vi "gu_list_folder.vi"(8 "error in":errorcluster, 10 "Encoded Match":T1, 11 "Encoded String":T1) -> (0 "error out":errorcluster, 2 "Encoded Folders":T1[](array[typedef]), 3 "Encoded Files":T1[](array[typedef]))   [LabVIEW 2020, in "G-Unicode.lvlib"]
uses:
  G-Unicode.lvlib
  Types/Encoded UTF-8 String.ctl
  lib/g_unicode_32.dll
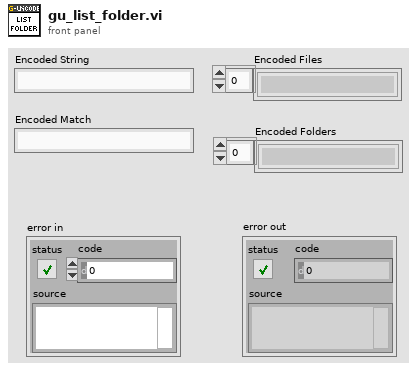
[diagram p1: front panel]
types:
  T1 = typedef "G-Unicode.lvlib/Encoded UTF-8 String.ctl" = string
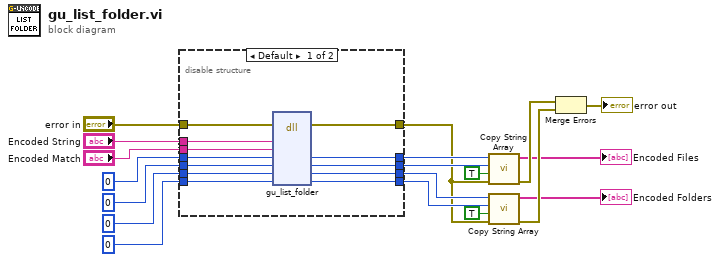
[diagram p0: block diagram]
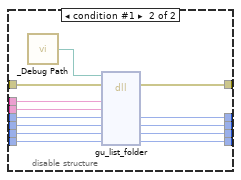
[diagram p2: hidden frame]
diagram:
  n1 = disable-structure shown="Default" {
    disable-tunnel: "Encoded String" -> [w31 w44]
    disable-tunnel: "error in" -> [w30 w43]
    disable-tunnel: [w29 w42] -> w9
    disable-tunnel: i64 0 ("files") -> [w28 w41]
    disable-tunnel: 0 ("num_files") -> [w27 w40]
    disable-tunnel: i64 0 ("folders") -> [w26 w39]
    disable-tunnel: 0 ("num_folders") -> [w25 w38]
    disable-tunnel: [w24 w37] -> w15
    disable-tunnel: [w23 w36] -> w14
    disable-tunnel: [w22 w35] -> w13
    disable-tunnel: [w21 w34] -> w12
    disable-tunnel: "Encoded Match" -> [w20 w32]
    frame condition #0 (active) {
      n2 = dll-call lib="C:/github/dataflowg/g-unicode/src/LabVIEW/G-Unicode/lib/g_unicode_*.*" fn="gu_list_folder"(error in=w30, "path"=w31, "match"=w20, "files"=w28, "num_files"=w27, "folders"=w26, "num_folders"=w25) -> (error out=w29:errorcluster, "files"=w24:i64, "num_files"=w23:i32, "folders"=w22:i64, "num_folders"=w21:i32)  [unwired: 5 in, 1 out]
    }
    frame condition #1 {
      n3 = call "_Debug Path.vi"() -> ("Debug Path"=w33:path)
      n4 = dll-call lib="?" fn="gu_list_folder"(path in=w33, error in=w43, "path"=w44, "match"=w32, "files"=w41, "num_files"=w40, "folders"=w39, "num_folders"=w38) -> (error out=w42:errorcluster, "files"=w37:i64, "num_files"=w36:i32, "folders"=w35:i64, "num_folders"=w34:i32)  [unwired: 4 in, 1 out]
    }
  }
  n5 = call "Copy String Array.vi"("error in"=w9, "free (F)"=TRUE, "size"=w14, "pointer"=w15) -> ("error out"=w8:errorcluster, "Strings"=→"Encoded Files":string[])  [unwired: 6 in]
  n6 = call "Copy String Array.vi"("error in"=w9, "free (F)"=TRUE, "size"=w12, "pointer"=w13) -> ("error out"=w7:errorcluster, "Strings"=→"Encoded Folders":string[])  [unwired: 6 in]
  n7 = Merge Errors(w8, w7) -> (→"error out":errorcluster)
